vi "ke622x_2182a_setdelta.vi"(0 "622x VISA":refnum<visa-resource-name>="GPIB0::12::INSTR", 1 "range /V":dbl=0.01 min=0.0 max=100.0, 5 "compliance abort":bool, 7 "DMM auto range":bool=TRUE, 9 "current /A":dbl=0.0001 min=0.0 max=0.1, 11 "error in (no error)":errorcluster caption="entrée d'erreur (pas d'erreur)", 12 "compliance /V":dbl=10.0 min=0.009999999776482582 max=42.0) -> (4 "622x out":refnum<visa-resource-name>="GPIB0::12::INSTR", 15 "error out":errorcluster caption="sortie d'erreur")   [LabVIEW 2018]
uses:
  <instrlib>/Keithley 622x LV 2009/Keithley 622x.lvlib
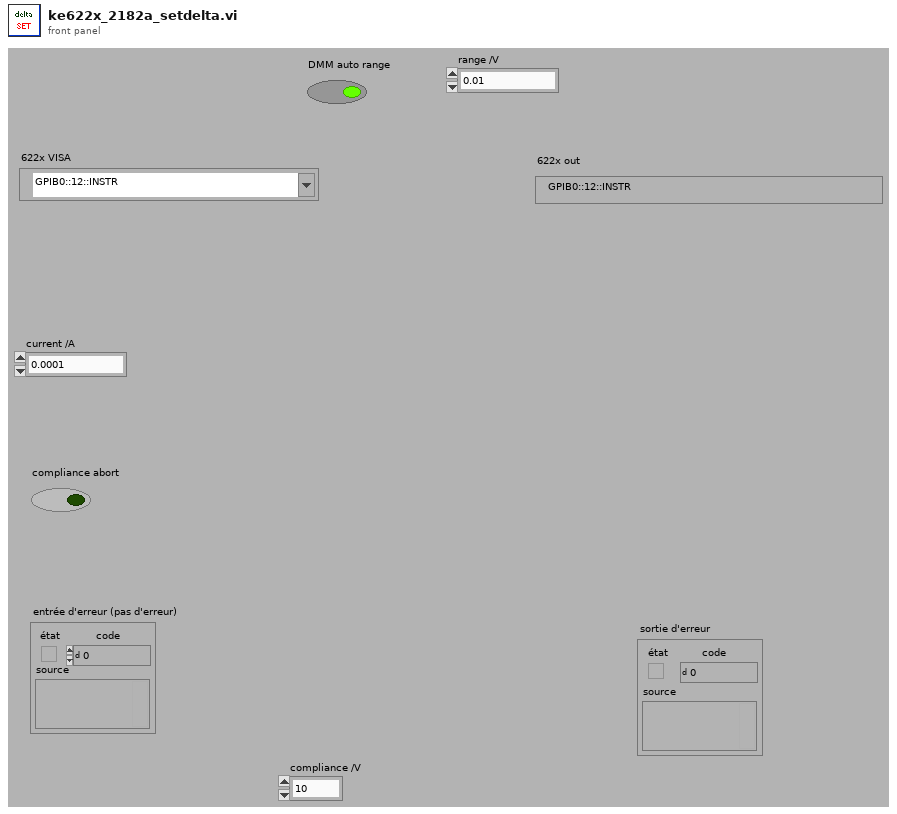
[diagram p1: front panel]
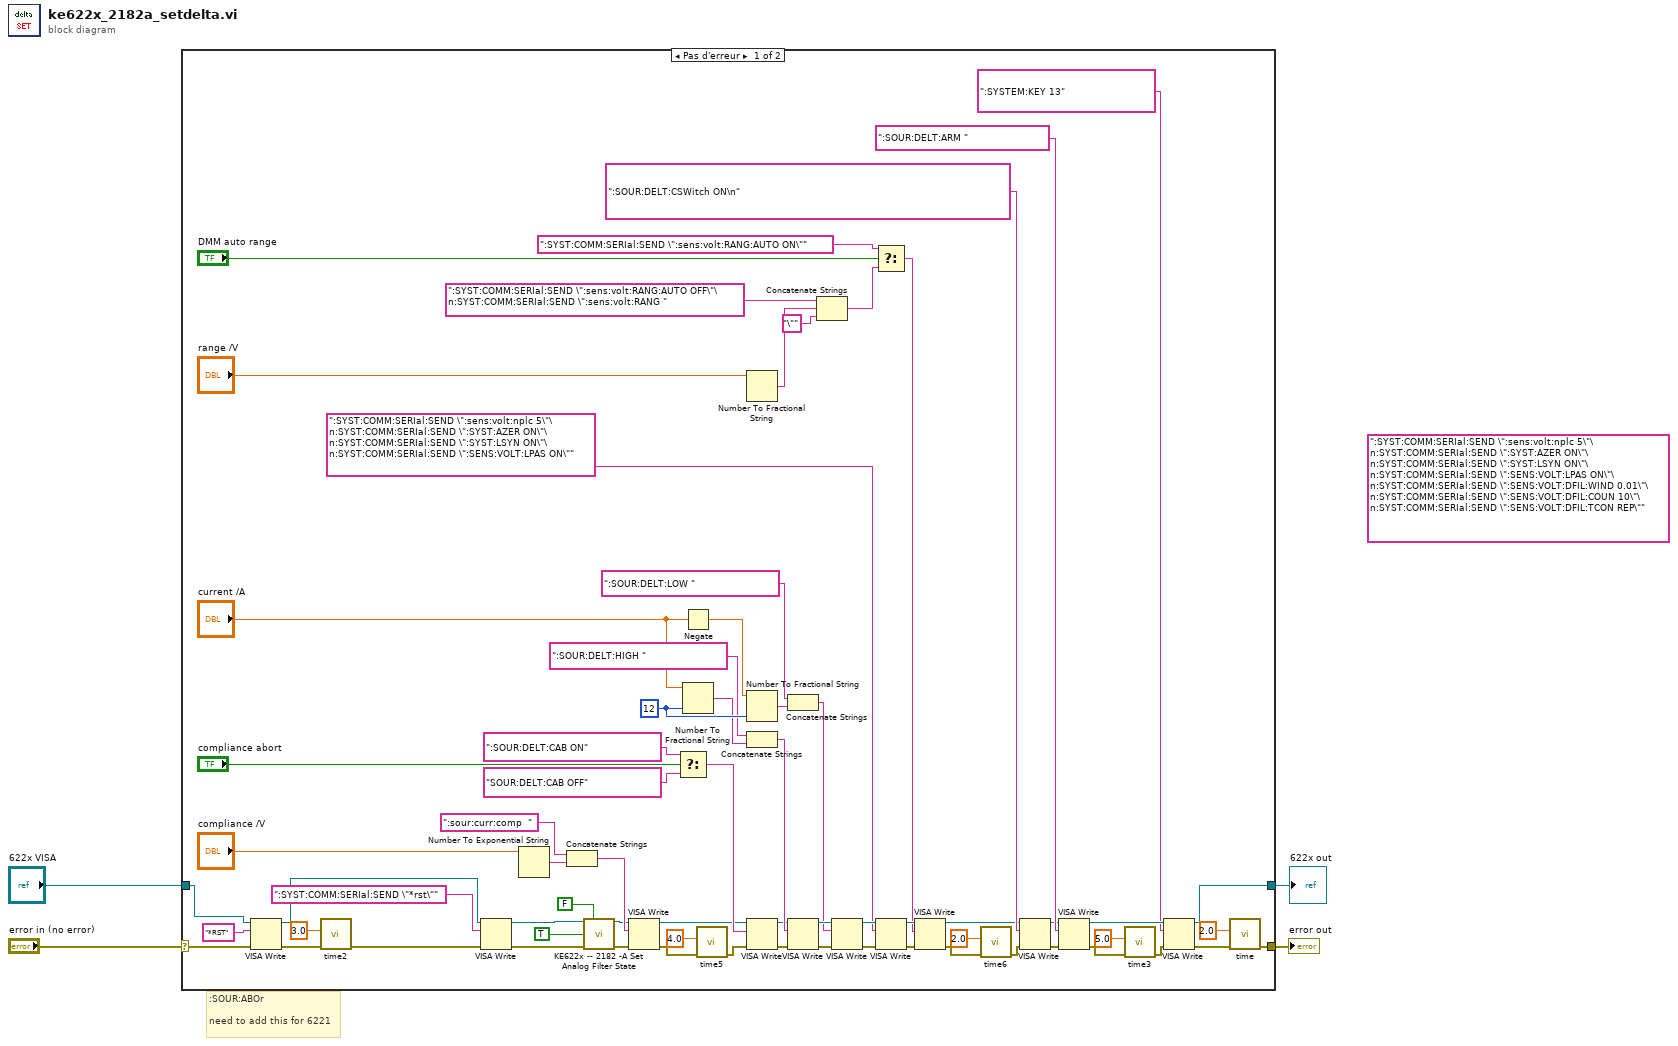
[diagram p0: block diagram]
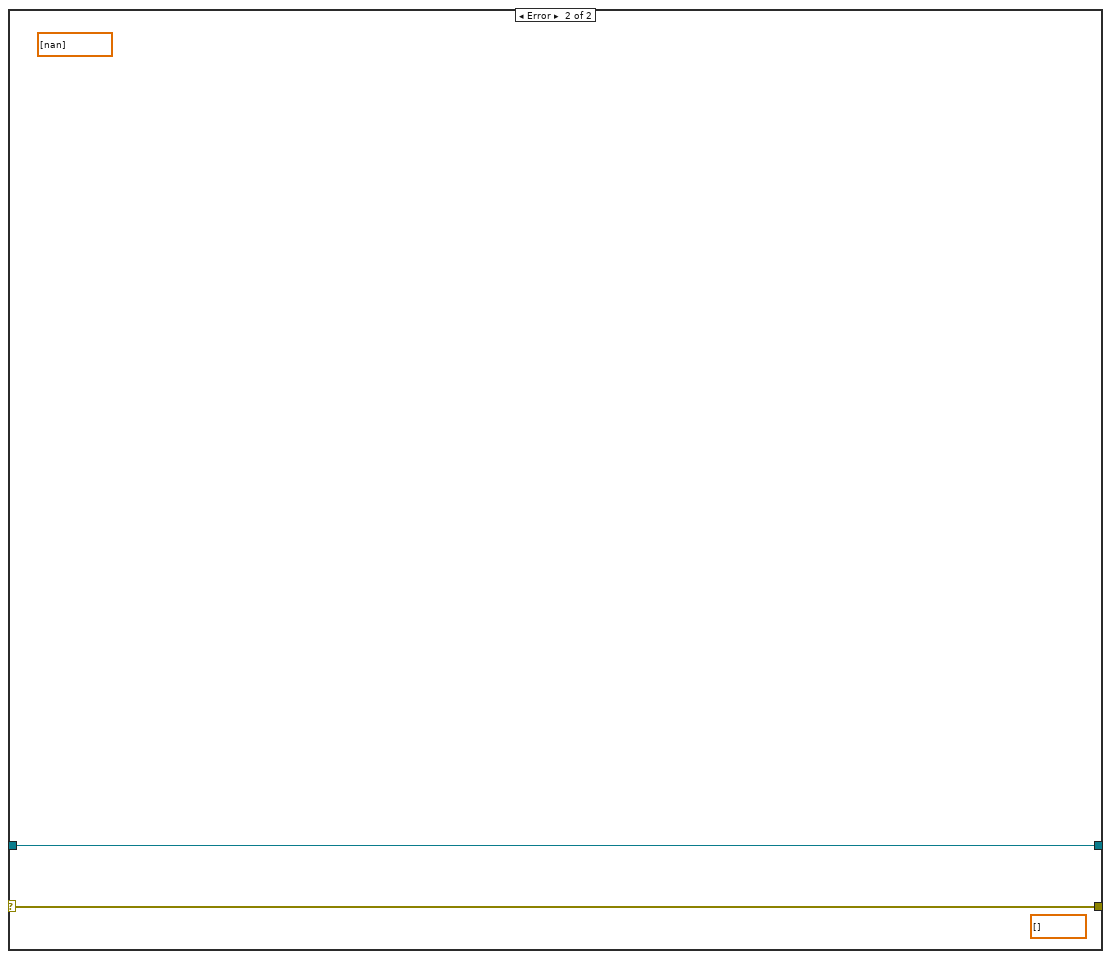
[diagram p2: hidden frame]
diagram:
  (unwired) ":SYST:COMM:SERIal:SEND \":sens:volt:nplc 5\"\n:SYST:COMM:SERIal:SEND \":SYST:AZER ON\"\n:SYST:COMM:SERIal:SEND \":SYST:LSYN ON\"\n:SYST:COMM:SERIal:SEND \":SENS:VOLT:LPAS ON\"\n:SYST:COMM:SERIal:SEND \":SENS:VOLT:DFIL:WIND 0.01\"\n:SYST:COMM:SERIal:SEND \":SENS:VOLT:DFIL:COUN 10\"\n:SYST:COMM:SERIal:SEND \":SENS:VOLT:DFIL:TCON REP\"" ("buffer à écrire")
  # ":SOUR:ABOr\n\nneed to add this for 6221"
  n1 = case shown="Pas d'erreur" "error in (no error)" {
    selector: "error in (no error)" -> [w38 w75]
    tunnel: [w34 w75] -> w3
    tunnel: "622x VISA" -> [w37 w74]
    tunnel: [w32 w74] -> w1
    frame No Error {
      w71 = i16 12 ("précision (6)")
      n2 = VISA Write(VISA resource name=w37, write buffer="*RST" ("buffer d'écriture"), error in (no error)=w38) -> (VISA resource name out=w7:refnum<visa-resource-name>, error out=w29:errorcluster)  [unwired: 1 out]
      n3 = call "time2"("error in (no error)"=w29, "Delay Time (s)"=3.0) -> ("error out"=w6:errorcluster)  [unwired: 9 out]
      n4 = VISA Write(VISA resource name=w7, write buffer=":SYST:COMM:SERIal:SEND \"*rst\"" ("buffer à écrire"), error in (no error)=w6) -> (VISA resource name out=w18:refnum<visa-resource-name>, error out=w17:errorcluster)  [unwired: 1 out]
      n5 = Number To Exponential String(number="compliance /V") -> (E-format string=w22:string)  [unwired: 3 out]
      n6 = Concatenate Strings(":sour:curr:comp  " ("buffer à écrire"), w22) -> (w23:string)
      n7 = call <instrlib>:"KE622x -- 2182 -A Set Analog Filter State.vi"("622x Resource In"=w18, "Check For SCPI Errors? (T)"=FALSE, "Enable Analog Filter?"=TRUE, "error in (no error)"=w17) -> ("622x Resource Out (dupl)"=w15:refnum<visa-resource-name>, "error out"=w16:errorcluster)  [unwired: 10 in]
      n8 = VISA Write(VISA resource name=w15, write buffer=w23, error in (no error)=w16) -> (VISA resource name out=w20:refnum<visa-resource-name>, error out=w19:errorcluster)  [unwired: 1 out]
      n9 = Select(t=":SOUR:DELT:CAB ON", s="compliance abort", f="SOUR:DELT:CAB OFF") -> (s? t:f=w57:string)
      n10 = Negate(x="current /A") -> (-x=w12:dbl)
      n11 = Number To Fractional String(number="current /A", precision (6)=w71) -> (F-format string=w69:string)  [unwired: 2 out]
      n12 = call "time5"("error in (no error)"=w19, "Delay Time (s)"=4.0) -> ("error out"=w26:errorcluster)  [unwired: 9 out]
      n13 = Number To Fractional String(number="range /V") -> (F-format string=w48:string)  [unwired: 3 out]
      n14 = Number To Fractional String(number=w12, precision (6)=w71) -> (F-format string=w66:string)  [unwired: 2 out]
      n15 = Concatenate Strings(":SOUR:DELT:HIGH ", w69) -> (w68:string)
      n16 = VISA Write(VISA resource name=w20, write buffer=w57, error in (no error)=w26) -> (VISA resource name out=w59:refnum<visa-resource-name>, error out=w58:errorcluster)  [unwired: 1 out]
      n17 = Concatenate Strings(":SOUR:DELT:LOW ", w66) -> (w65:string)
      n18 = VISA Write(VISA resource name=w59, write buffer=w68, error in (no error)=w58) -> (VISA resource name out=w73:refnum<visa-resource-name>, error out=w72:errorcluster)  [unwired: 1 out]
      n19 = Concatenate Strings(":SYST:COMM:SERIal:SEND \":sens:volt:RANG:AUTO OFF\"\n:SYST:COMM:SERIal:SEND \":sens:volt:RANG " ("buffer à écrire"), w48, "\"" ("buffer à écrire")) -> (w39:string)
      n20 = VISA Write(VISA resource name=w73, write buffer=w65, error in (no error)=w72) -> (VISA resource name out=w28:refnum<visa-resource-name>, error out=w27:errorcluster)  [unwired: 1 out]
      n21 = Select(t=":SYST:COMM:SERIal:SEND \":sens:volt:RANG:AUTO ON\"" ("buffer à écrire"), s="DMM auto range", f=w39) -> (s? t:f=w42:string)
      n22 = VISA Write(VISA resource name=w28, write buffer=":SYST:COMM:SERIal:SEND \":sens:volt:nplc 5\"\n:SYST:COMM:SERIal:SEND \":SYST:AZER ON\"\n:SYST:COMM:SERIal:SEND \":SYST:LSYN ON\"\n:SYST:COMM:SERIal:SEND \":SENS:VOLT:LPAS ON\"" ("buffer à écrire"), error in (no error)=w27) -> (VISA resource name out=w45:refnum<visa-resource-name>, error out=w43:errorcluster)  [unwired: 1 out]
      n23 = VISA Write(VISA resource name=w45, write buffer=w42, error in (no error)=w43) -> (VISA resource name out=w44:refnum<visa-resource-name>, error out=w10:errorcluster)  [unwired: 1 out]
      n24 = call "time6"("error in (no error)"=w10, "Delay Time (s)"=2.0) -> ("error out"=w9:errorcluster)  [unwired: 9 out]
      n25 = VISA Write(VISA resource name=w44, write buffer=":SOUR:DELT:CSWitch ON\n", error in (no error)=w9) -> (VISA resource name out=w53:refnum<visa-resource-name>, error out=w52:errorcluster)  [unwired: 1 out]
      n26 = VISA Write(VISA resource name=w53, write buffer=":SOUR:DELT:ARM ", error in (no error)=w52) -> (VISA resource name out=w63:refnum<visa-resource-name>, error out=w51:errorcluster)  [unwired: 1 out]
      n27 = call "time3"("error in (no error)"=w51, "Delay Time (s)"=5.0) -> ("error out"=w50:errorcluster)  [unwired: 9 out]
      n28 = VISA Write(VISA resource name=w63, write buffer=":SYSTEM:KEY 13", error in (no error)=w50) -> (VISA resource name out=w32:refnum<visa-resource-name>, error out=w35:errorcluster)  [unwired: 1 out]
      n29 = call "time"("error in (no error)"=w35, "Delay Time (s)"=2.0) -> ("error out"=w34:errorcluster)  [unwired: 9 out]
    }
    frame Error {
      (unwired) dbl[] []
      (unwired) dbl[] [nan]
    }
  }
  "error out" <- w3
  "622x out" <- w1
